vi "Get PSU Field.vi"(8 "error in (no error)":errorcluster, 11 "Instrument.Oxford1820 in":refnum<class "Instrument.Oxford1820.lvclass">) -> (0 "error out":errorcluster, 2 "PSU Field (T)":dbl, 3 "Instrument.Oxford1820 out":refnum<class "Instrument.Oxford1820.lvclass">)   [LabVIEW 2016, in "Instrument.Oxford1820.lvclass"]
uses:
  Instrument.Oxford1820.lvclass
  Typedefs/Instrument.Oxford1820.Commands-enum.ctl
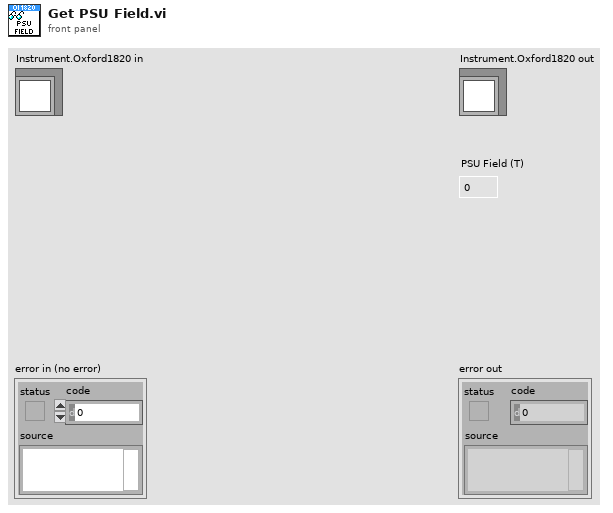
[diagram p1: front panel]
types:
  T1 = typedef "Instrument.Oxford1820.lvclass/Instrument.Oxford1820.Commands-enum.ctl" = enum16{"setAction", "setTarget", "setSwitchHeat", "setLambda", "setFillMode", "setNeedleValve", "setMagnetField", "getStatus", "getTarget", "getSwitchHeat", "getPSUField", "getMagnetField"}
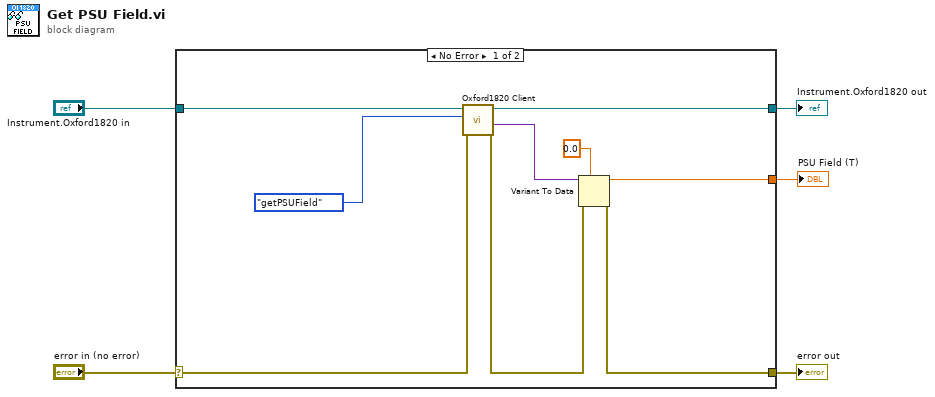
[diagram p0: block diagram]
diagram:
  n1 = case shown="No Error" "error in (no error)" {
    selector: "error in (no error)" -> [w11 w16]
    tunnel: [w7 w16] -> w4
    tunnel: [w12 w15] -> w2
    tunnel: "Instrument.Oxford1820 in" -> [w13 w15]
    tunnel: [w6 _] -> w1
    frame No Error {
      n2 = call "Oxford1820 Client.vi"("error in (no error)"=w11, "Commands"=Instrument.Oxford1820.Commands-enum."getPSUField", "Instrument.1820 in"=w13) -> ("error out"=w8:errorcluster, "Data out"=w10:variant, "Instrument.1820 out"=w12:refnum<class "Instrument.Oxford1820.lvclass">)  [unwired: 6 in]
      n3 = Variant To Data(error in=w8, type=0.0, Variant=w10) -> (data=w6:dbl, error out=w7:errorcluster)
    }
    frame Error {
    }
  }
  "error out" <- w4
  "Instrument.Oxford1820 out" <- w2
  "PSU Field (T)" <- w1
